vi "FormatColor.vi"(1 "color":u32(colorbox)) -> (0 "value":string)   [LabVIEW 2014, in "PythonConfiguration.lvclass"]
uses:
  PythonConfiguration.lvclass
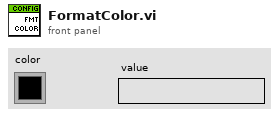
[diagram p1: front panel]
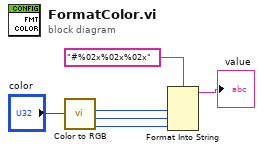
[diagram p0: block diagram]
diagram:
  n1 = call <vilib>:"Color to RGB.vi"("Color"="color") -> ("R"=w3:u8, "G"=w2:u8, "B"=w1:u8)  [unwired: 1 out]
  n2 = Format Into String(format string="#%02x%02x%02x", w3, w2, w1) -> (resulting string=→"value":string)  [unwired: 2 in, 1 out]
